vi "Add Customer with Phone.vi"(7 "Time scale [ms]":u32=5000, 8 "error in (no error)":errorcluster, 10 "Name":string, 11 "Coffee Shop in":refnum<class "Coffee Shop.lvclass">) -> (0 "error out":errorcluster, 3 "Coffee Shop out":refnum<class "Coffee Shop.lvclass">)   [LabVIEW 2020, in "Coffee Shop.lvclass"]
uses:
  Coffee Shop.lvclass
  C:/Program Files (x86)/National Instruments/LabVIEW 2020/vi.lib/Astemes/Triarc Framework/Process/Process.lvclass
  People/Customers/Customer With Phone/Customer With Phone.lvclass
  C:/git/astemes-triarc-examples/source/Coffee Shop/Processes/People/Person/Person.lvclass
  C:/git/astemes-triarc-examples/source/Coffee Shop/Processes/People/Customers/Customer/Customer.lvclass
  <vilib>/Astemes/Triarc Framework/Process/Process.lvclass/Process.ctl
  People/Person/Person.lvclass/Person.ctl
  <vilib>/Astemes/Triarc Framework/Process/Private/SubVIs/Handle Debug Data.vi
  <vilib>/Astemes/Triarc Framework/Logging/Log Debug.vi
  <vilib>/AdvancedString/1D String Array to Delimited String.vi
  <vilib>/Utility/High Resolution Relative Seconds.vi
  People/Person/Person.lvclass
  <vilib>/Astemes/Triarc Framework/Process/Public/Lifecycle/Get Lifecycle State.vi
  <vilib>/Astemes/Triarc Framework/Process/Public/Read Name.vi
  <vilib>/Astemes/Triarc Framework/Callback/Callback.lvclass
  <vilib>/Astemes/Triarc Framework/Process/Process.lvclass
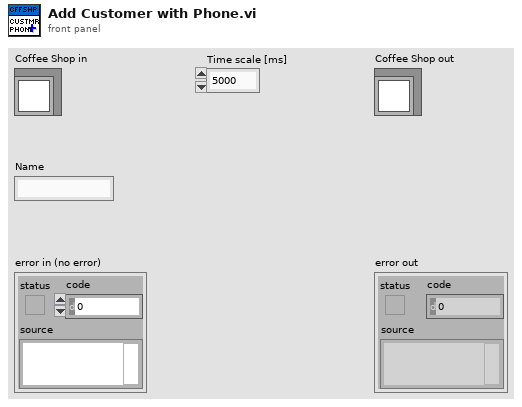
[diagram p1: front panel]
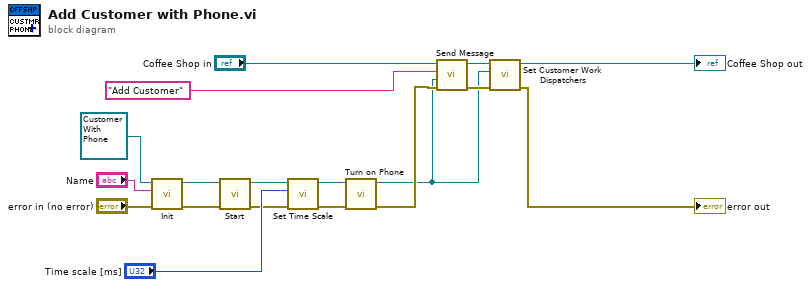
[diagram p0: block diagram]
diagram:
  n1 = call-dynamic "Init.vi"("error in (no error)"="error in (no error)", "Name"="Name", "View In"=refnum<class "Customer With Phone.lvclass"> refnum ("Customer With Phone.lvclass")) -> ("error out"=w12:errorcluster, "View Out"=w2:refnum<class "Customer With Phone.lvclass">)  [unwired: 7 in]
  n2 = call <vilib>:"Start.vi"("error in (no error)"=w12, "Process In"=w2) -> ("error out"=w3:errorcluster, "Process Out"=w1:refnum<class "Customer With Phone.lvclass">)  [unwired: 7 in, 1 out]
  n3 = call "Set Time Scale.vi"("TRIARC_ERROR_IN"=w3, "Time Scale [ms]"="Time scale [ms]", "Person In"=w1) -> ("TRIARC_ERROR_OUT"=w8:errorcluster, "Person Out"=w5:refnum<class "Customer With Phone.lvclass">)  [unwired: 7 in]
  n4 = call "Turn on Phone.vi"("error in (no error)"=w8, "Customer With Phone In"=w5) -> ("error out"=w6:errorcluster, "Customer With Phone Out"=w4:refnum<class "Customer With Phone.lvclass">)  [unwired: 8 in]
  n5 = call <vilib>:"Send Message.vi"("error in (no error)"=w6, "Message Data"=w4, "Message"="Add Customer", "Process In"="Coffee Shop in") -> ("error out"=w18:errorcluster, "Process Out"=w11:refnum<class "Coffee Shop.lvclass">)  [unwired: 6 in]
  n6 = call "Set Customer Work Dispatchers.vi"("error in (no error)"=w18, "Customer"=w4, "Coffee Shop In"=w11) -> ("error out"=→"error out":errorcluster, "Coffee Shop Out"=→"Coffee Shop out":refnum<class "Coffee Shop.lvclass">)  [unwired: 7 in]
